vi "algo 4.vi"(0 "Range (Threshold 1)":cluster{"Lower value":sgl, "Upper value":sgl}={"Lower value"=0.0, "Upper value"=47.0}, 7 "error in":errorcluster) -> (20 "Circles (Shape Detection 1)":T2(array[cluster]) {"Position"."Y" format="%.2f"; "Position"."X" format="%.2f"}, 22 "Number of Matches (Shape Detection 1)":i32, 27 "error out":errorcluster)   [LabVIEW 2015]
uses:
  <vilib>/userdefined/High Color/IMAQdx.ctl
  <vilib>/vision/NI_Vision_Development_Module.lvlib
  <vilib>/vision/driver/NI_Vision_Acquisition_Software.lvlib
panel:
  out "FramePeriod":u32
  in  "stop":bool
  out "Image Out":T1(plugin-control)
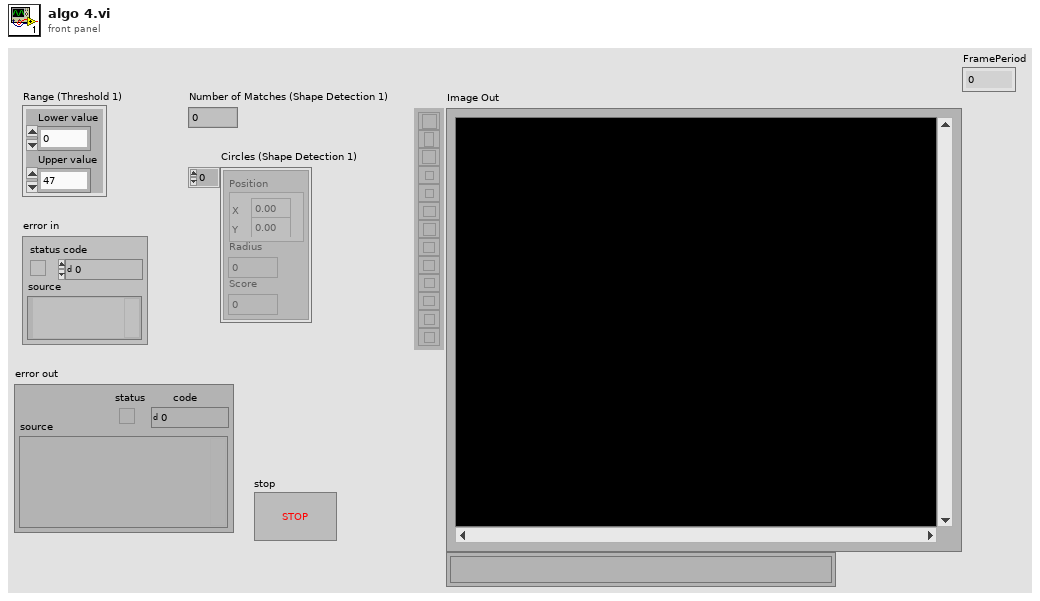
[diagram p1: front panel]
types:
  T1 = typedef "IMAQ Image.ctl" = refnum<image>
  T2 = cluster{"Position":cluster{"X":sgl, "Y":sgl}, "Radius":dbl, "Score":dbl}[]
  T3 = typedef "IMAQdx.ctl" = refnum<k21>
  T4 = cluster{"Left":i32, "Top":i32, "Right":i32, "Bottom":i32}
  T5 = cluster{"Extraction Mode":u32, "Edge Threshold":i32, "Edge Filter Size":u32, "Min Length":i32, "Row Search Step Size":i32, "Col Search Step Size":i32, "Max Endpoint Gap":i32, "Closed":bool, "Subpixel":bool}
  T6 = cluster{"Rotation":bool, "Scale":bool, "Occlusion":bool, "Range Settings":cluster{"Match Constraints":u32, "Min":dbl, "Max":dbl}[]}
  T7 = cluster{"Global Rectangle":i32[], "Contours":cluster{"ID":enum32{"External", "Internal"}, "Type":u32, "Coordinates":i32[]}[]}
  T8 = cluster{"Position":cluster{"X":sgl, "Y":sgl}, "Radius":dbl, "Score":dbl}
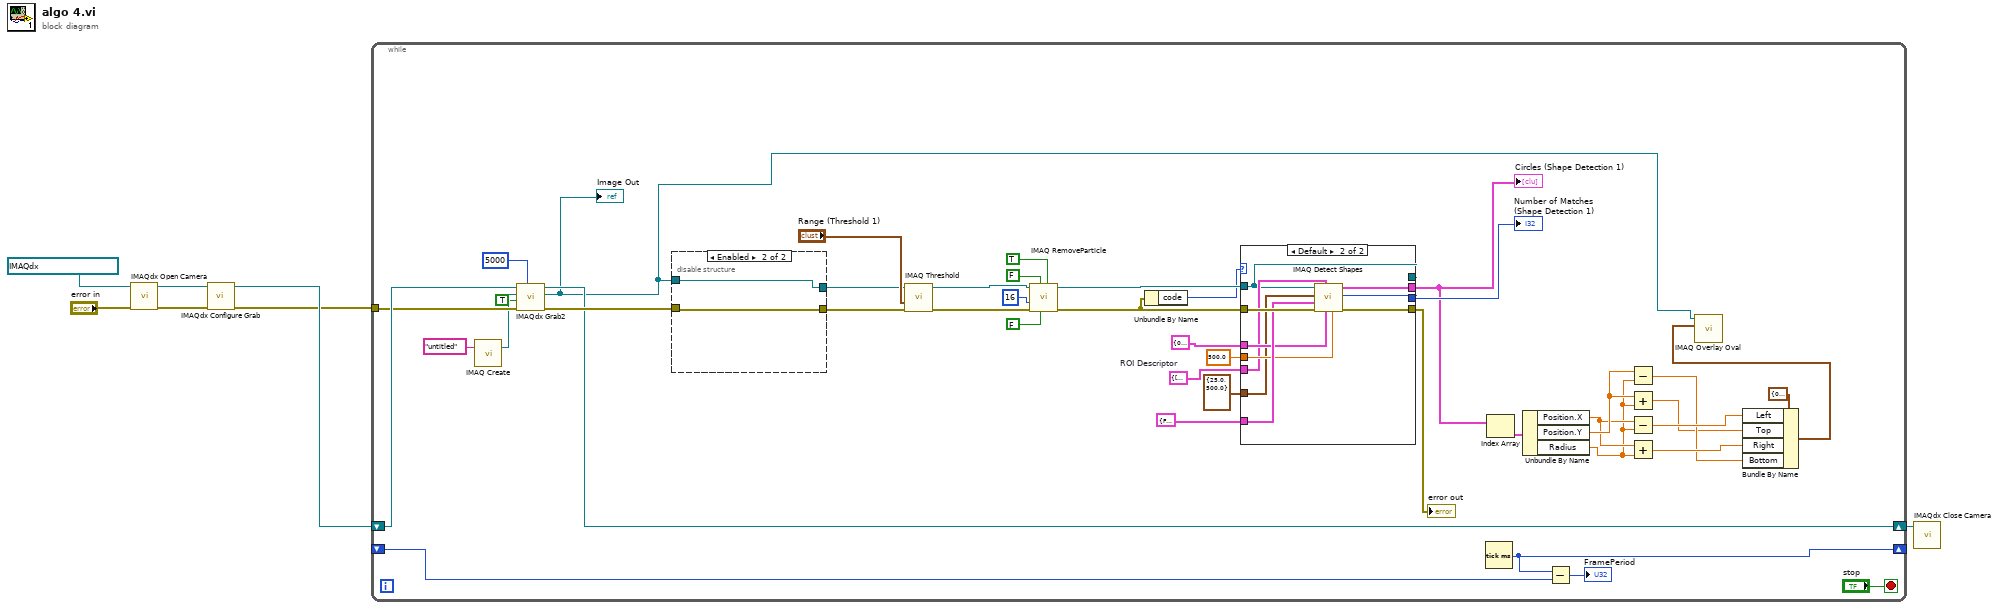
[diagram p0: block diagram]
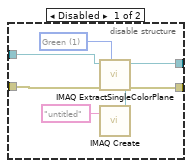
[diagram p2: hidden frame]
diagram:
  n1 = call <vilib>:"IMAQdx Open Camera.vi"("error in"="error in", "Session In"=T3 "acA1300-60gmNIR") -> ("error out"=w2:errorcluster, "Session Out"=w4:T3)  [unwired: 8 in]
  n2 = call <vilib>:"IMAQdx Configure Grab.vi"("error in"=w2, "Session In"=w4) -> ("error out"=w1:errorcluster, "Session Out"=w3:T3)  [unwired: 8 in]
  n3 = while {
    tunnel: w1 -> [w19]
    shift-right: [w9] -> w5
    shift-left: w3 -> [w20]
    shift-right: [w14] -> _
    shift-left: _ -> [w13]
    stop <- "stop" stop-if-true
    w36 = T7 {"Global Rectangle"=[20, 20, 1580, 649], "Contours"=[{"ID"=enum."External", "Type"=3, "Coordinates"=[20, 20, 1580, 649]}]}  # ROI Descriptor
    n4 = call "IMAQ Create"("Image Name"="untitled") -> ("New Image"=w18:T1)  [unwired: 4 in, 1 out]
    n5 = call <vilib>:"IMAQdx Grab2.vi"("Timeout (ms)"=5000, "error in"=w19, "Wait for Next Buffer? (Yes)"=TRUE, "Image In"=w18, "Session In"=w20) -> ("error out"=w17:errorcluster, "Image Out"=w8:T1, "Session Out"=w9:T3)  [unwired: 3 in, 1 out]
    "Image Out" <- w8
    n6 = disable-structure shown="Enabled" {
      disable-tunnel: [w56 w59] -> w49
      disable-tunnel: [w55 w58] -> w48
      disable-tunnel: w17 -> [w54 w58]
      disable-tunnel: w8 -> [w53 w59]
      frame Disabled {
        w57 = 1 items=["Red", "Green", "Blue", "Hue", "Saturation", "Luminance", "Value", "Intensity"] ("Color Plane")
        n7 = call "IMAQ Create"("Image Name"="untitled") -> ("New Image"=w51:T1)  [unwired: 4 in, 1 out]
        n8 = call "IMAQ ExtractSingleColorPlane"("Color Plane"=w57, "error in (no error)"=w54, "Image Dst"=w51, "Image Src"=w53) -> ("error out"=w55:errorcluster, "Image Dst Out"=w56:T1)  [unwired: 6 out]
      }
      frame Enabled {
      }
    }
    n9 = call "IMAQ Threshold"("error in (no error)"=w48, "Range"="Range (Threshold 1)", "Image Src"=w49) -> ("error out"=w42:errorcluster, "Image Dst Out"=w43:T1)  [unwired: 3 in, 4 out]
    n10 = call "IMAQ RemoveParticle"("Connectivity 4/8 (8)"=TRUE, "Low Pass/High Pass (Low)"=FALSE, "Square/Hexa (Square)"=FALSE, "error in (no error)"=w42, "Number of Erosion"=16, "Image Src"=w43) -> ("error out"=w34:errorcluster, "Image Dst Out"=w35:T1)  [unwired: 1 in, 3 out]
    n11 = Unbundle By Name(w34) -> ("code"=w33:i32)
    n12 = case shown="Default" w33 {
      tunnel: w34 -> [_ w70]
      tunnel: [_ w69] -> w41
      tunnel: T6 {"Rotation"=FALSE, "Scale"=FALSE, "Occlusion"=TRUE, "Range Settings"=[{"Match Constraints"=2, "Min"=0.0, "Max"=50.0}]} ("Match Options") -> [_ w68]
      tunnel: T5 {"Extraction Mode"=0, "Edge Threshold"=1, "Edge Filter Size"=1, "Min Length"=40, "Row Search Step Size"=15, "Col Search Step Size"=15, "Max Endpoint Gap"=10, "Closed"=FALSE, "Subpixel"=FALSE} ("Curve Parameters") -> [_ w67]
      tunnel: 500.0 ("Minimum match score") -> [_ w66]
      tunnel: cluster{"Min Radius":dbl, "Max Radius":dbl} {"Min Radius"=25.0, "Max Radius"=500.0} ("Circle Descriptor") -> [_ w65]
      tunnel: w36 -> [_ w64]
      tunnel: [_ w63] -> w26
      tunnel: w35 -> [w60 w61]
      tunnel: [_ w62] -> w25
      tunnel: [w60 w61] -> _
      frame -1074396199, -1074396198 {
        # "Discard Coordinate\nSystem Error"
      }
      frame Default {
        n13 = call-poly "IMAQ Detect Shapes"("Minimum match score"=w66, "Curve Parameters"=w67, "ROI Descriptor"=w64, "error in (no error)"=w70, "Match Options"=w68, "Circle Descriptor"=w65, "Image"=w61) -> ("error out"=w62:errorcluster, "Number of Matches Returned"=w69:i32, "Circles"=w63:T2)  [unwired: 2 out]
      }
    }
    "Number of Matches (Shape Detection 1)" <- w41
    "Circles (Shape Detection 1)" <- w26
    "error out" <- w25
    n14 = Tick Count (ms)() -> (millisecond timer value=w14:u32)
    n15 = Index Array(array=w26) -> (element=w24:T8)  [unwired: 1 in]
    n16 = Unbundle By Name(w24) -> ("Position.X"=w22:sgl, "Position.Y"=w23:sgl, "Radius"=w21:dbl)
    n17 = Subtract(x=w14, y=w13) -> (x-y=→"FramePeriod":u32)
    n18 = Subtract(x=w23, y=w21) -> (x-y=w29:dbl)
    n19 = Add(x=w23, y=w21) -> (x+y=w28:dbl)
    n20 = Subtract(x=w22, y=w21) -> (x-y=w31:dbl)
    n21 = Add(x=w22, y=w21) -> (x+y=w30:dbl)
    n22 = Bundle By Name(cluster=T4 {"Left"=0, "Top"=0, "Right"=0, "Bottom"=0} ("Bounding Rectangle"), "Left"=w31, "Top"=w28, "Right"=w30, "Bottom"=w29) -> (w27:T4)
    n23 = call "IMAQ Overlay Oval"("Bounding Rectangle"=w27, "Image"=w8) -> ()  [unwired: 8 in, 2 out]
  }
  n24 = call <vilib>:"IMAQdx Close Camera.vi"("Session In"=w5) -> ()  [unwired: 10 in, 1 out]
